vi "Counter - Continuous Output.vi"() -> ()   [LabVIEW 2012, in "Waveform.lvclass"]
doc: "This example demonstrates how to continuously generate digital pulses using a counter output."
uses:
  Waveform.lvclass
  <vilib>/Utility/error.llb/DialogType.ctl
  <vilib>/DAQmx/write.llb/DAQmx Write (Analog Wfm 1Chan NSamp).vi
  <vilib>/DAQmx/create/channels.llb/DAQmx Create Channel (CO-Pulse Generation-Frequency).vi
  <vilib>/DAQmx/configure/timing.llb/DAQmx Timing (Implicit).vi
  <vilib>/DAQmx/create/channels.llb/DAQmx Create Channel (AO-Voltage-Basic).vi
  <vilib>/DAQmx/configure/timing.llb/DAQmx Timing (Sample Clock).vi
  <vilib>/DAQmx/configure/trigger.llb/DAQmx Start Trigger (Digital Edge).vi
  <vilib>/DAQmx/miscellaneous.llb/DAQmx Fill In Error Info.vi
  <resource>/objmgr/daqmx.rc
  <vilib>/measure/NI_MABase.lvlib
panel:
  in  "Amplitude":dbl=1.0 format="%0.2p"
  in  "Signal Type":T1(ring)
  in  "HSYNC":i32=1000
  in  "Frame Rate":dbl=10000.0 caption="frame Rate" format="%0.2f"
  in  "Minimum Value":dbl=-10.0 format="%0.2f"
  in  "Maximum Value":dbl=10.0 format="%0.2f"
  in  "Physical Channels":tag="Dev1/ao0"
  in  "error in":errorcluster
  out "Actual Duty Cycle":dbl
  out "Actual Frequency":dbl
  in  "Duty Cycle":dbl=0.5 format="%.6f"
  in  "Frequency":dbl=1.0 format="%.6f"
  in  "Output Terminal":tag="/Dev1/PFI12"
  in  "Trigger Type":T2(tab)
  in  "Edge":i32(ring)=10280 items=["Rising"=10280, "Falling"=10171]
  in  "Digital Trigger Source":tag
  in  "Pause When":i32(ring)=10192 items=["High"=10192, "Low"=10214]
  in  "Pause Trigger Source":tag
  in  "Stop":bool
  in  "Counter":tag="Dev1/ctr0"
  # "Channel Settings"
  # "Trigger Settings"
  # "To configure and use a trigger you must have the necessary tab selected above."
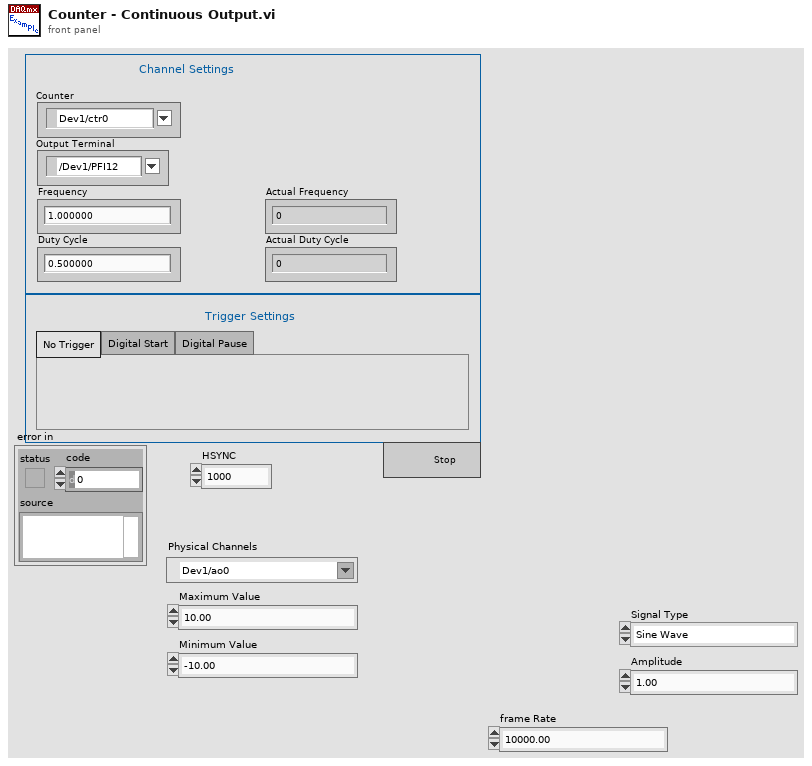
[diagram p1: front panel]
types:
  T1 = enum16{"Sine Wave", "Triangle Wave", "Square Wave", "Sawtooth Wave"}
  T2 = enum32{"No Trigger", "Digital Start", "Digital Pause"}
  T3 = typedef "DialogType.ctl" = u16
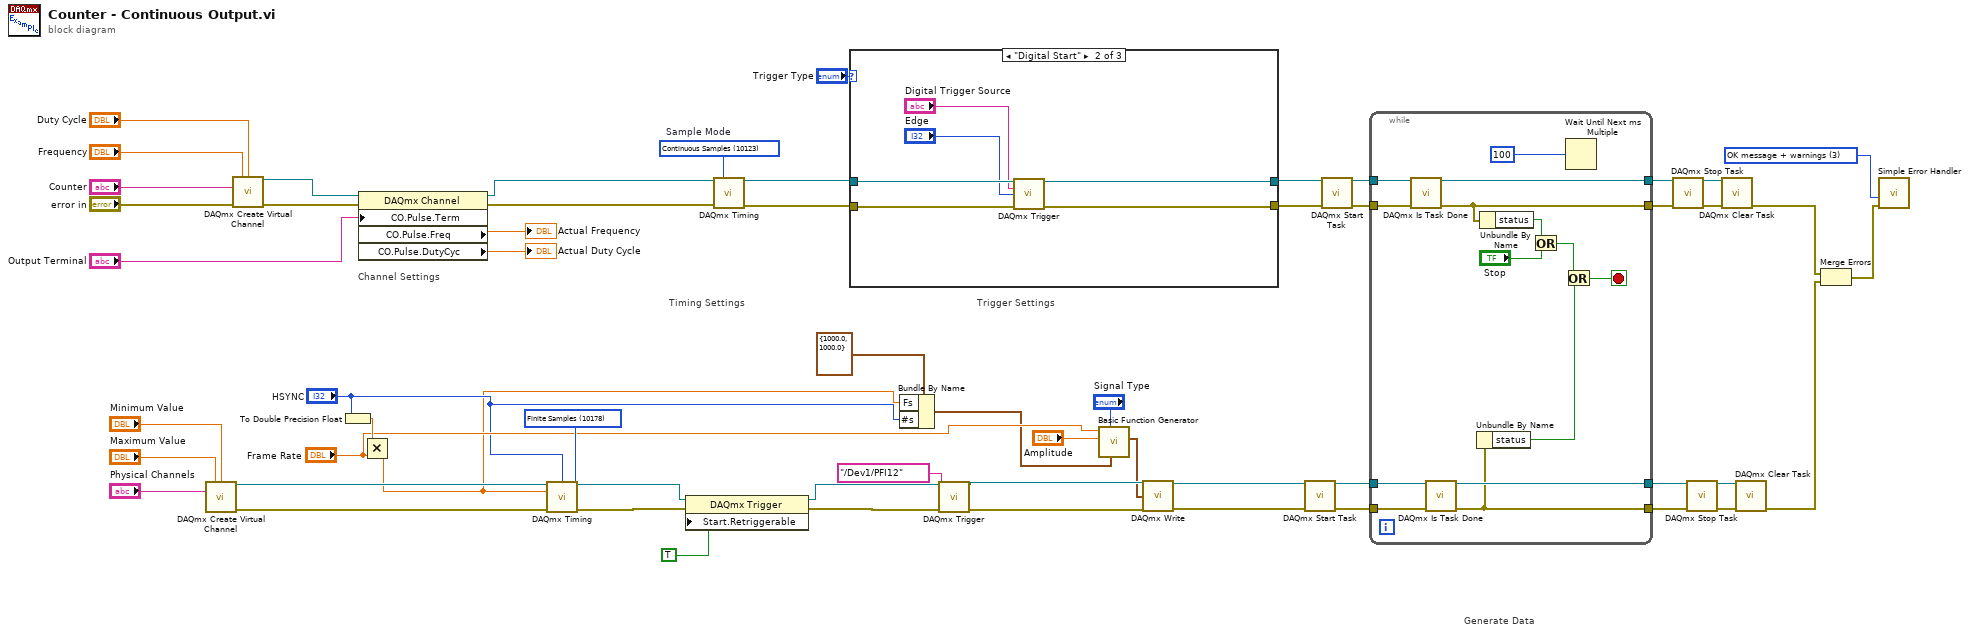
[diagram p0: block diagram]
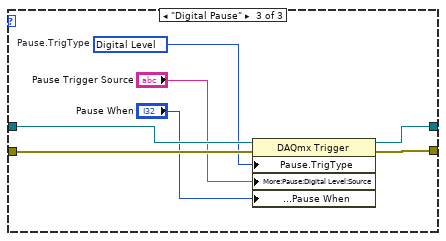
[diagram p3: hidden frame]
diagram:
  w29 = 10178 items=["Finite Samples"=10178, "Continuous Samples"=10123] ("sample mode")
  w36 = T3 3 items=["no dialog", "OK message", "continue or stop message", "OK message + warnings", "continue/stop + warnings"] ("type of dialog (OK msg:1)")
  w58 = 10123 items=["Finite Samples"=10178, "Continuous Samples"=10123, "Hardware Timed Single Point"=12522]  # Sample Mode
  # "Generate Data"
  # "Trigger Settings"
  # "Timing Settings"
  # "Channel Settings"
  n1 = call-poly <vilib>:"DAQmx Create Virtual Channel.vi"("maximum value"="Maximum Value", "minimum value"="Minimum Value", "physical channels"="Physical Channels") -> ("task out"=w32:refnum<k21>, "error out"=w28:errorcluster)  [unwired: 11 in]
  n2 = call-poly <vilib>:"DAQmx Create Virtual Channel.vi"("frequency"="Frequency", "duty cycle"="Duty Cycle", "counter"="Counter", "error in"="error in") -> ("task out"=w49:refnum<k21>, "error out"=w48:errorcluster)  [unwired: 10 in]
  n3 = To Double Precision Float(number="HSYNC") -> (double precision float=w33:dbl)
  n4 = property class="DAQmx Channel"(reference=w49, error in=w48, "CO.Pulse.Term"="Output Terminal") -> (reference out=w45:refnum<k21>, error out=w46:errorcluster, "CO.Pulse.Freq"=→"Actual Frequency":dbl, "CO.Pulse.DutyCyc"=→"Actual Duty Cycle":dbl)
  n5 = Multiply(x=w33, y="Frame Rate") -> (x*y=w7:dbl)
  n6 = call-poly <vilib>:"DAQmx Timing.vi"("task/channels in"=w32, "sample mode"=w29, "samples per channel"="HSYNC", "rate"=w7, "error in"=w28) -> ("task out"=w4:refnum<k21>, "error out"=w2:errorcluster)  [unwired: 9 in]
  n7 = property class="DAQmx Trigger"(reference=w4, error in=w2, "Start.Retriggerable"=TRUE) -> (reference out=w3:refnum<k21>, error out=w1:errorcluster)
  n8 = call-poly <vilib>:"DAQmx Timing.vi"("task/channels in"=w45, "sample mode"=w58, "error in"=w46) -> ("task out"=w53:refnum<k21>, "error out"=w52:errorcluster)  [unwired: 11 in]
  n9 = case shown="\"Digital Start\"" "Trigger Type" {
    tunnel: w53 -> [w60 w66 w73]
    tunnel: w52 -> [w59 w65 w70]
    tunnel: [w60 w64 w72] -> w50
    tunnel: [w59 w63 w71] -> w51
    frame "No Trigger", Default {
    }
    frame "Digital Start" {
      n10 = call-poly <vilib>:"DAQmx Trigger.vi"("task/channels in"=w66, "source"="Digital Trigger Source", "edge"="Edge", "error in"=w65) -> ("task out"=w64:refnum<k21>, "error out"=w63:errorcluster)  [unwired: 10 in]
    }
    frame "Digital Pause" {
      w69 = 10152 items=["Analog Level"=10101, "Analog Window"=10103, "Digital Level"=10152, "Digital Pattern"=10398, "None"=10230]  # Pause.TrigType
      n11 = property class="DAQmx Trigger"(reference=w73, error in=w70, "Pause.TrigType"=w69, "More:Pause:Digital Level:Source"="Pause Trigger Source", "More:Pause:Digital Level:Pause When"="Pause When") -> (reference out=w72:refnum<k21>, error out=w71:errorcluster)
    }
  }
  n12 = Bundle By Name(cluster=cluster{"Fs":dbl, "#s":dbl} {"Fs"=1000.0, "#s"=1000.0} ("sampling info"), "Fs"=w7, "#s"="HSYNC") -> (w6:cluster{"Fs":dbl, "#s":dbl})
  n13 = call-poly <vilib>:"DAQmx Trigger.vi"("task/channels in"=w3, "source"=tag "/Dev1/PFI12", "error in"=w1) -> ("task out"=w24:refnum<k21>, "error out"=w23:errorcluster)  [unwired: 11 in]
  n14 = call <vilib>:"Basic Function Generator.vi"("sampling info"=w6, "signal type"="Signal Type", "amplitude"="Amplitude", "frequency"="Frame Rate") -> ("signal out"=w22:waveform(dbl))  [unwired: 5 in, 2 out]
  n15 = call-poly <vilib>:"DAQmx Write.vi"("task/channels in"=w24, "data"=w22, "error in"=w23) -> ("task out"=w21:refnum<k21>, "error out"=w20:errorcluster)  [unwired: 10 in, 1 out]
  n16 = call <vilib>:"DAQmx Start Task.vi"("task/channels in"=w21, "error in"=w20) -> ("task out"=w19:refnum<k21>, "error out"=w18:errorcluster)  [unwired: 12 in]
  n17 = call <vilib>:"DAQmx Start Task.vi"("task/channels in"=w50, "error in"=w51) -> ("task out"=w57:refnum<k21>, "error out"=w56:errorcluster)  [unwired: 12 in]
  n18 = while {
    tunnel: w57 -> [w87]
    tunnel: w56 -> [w86]
    tunnel: [w84] -> w37
    tunnel: [w85] -> w38
    tunnel: w19 -> [w80]
    tunnel: w18 -> [w79]
    tunnel: [w78] -> w15
    tunnel: [w74] -> w14
    stop <- w75 stop-if-true
    n19 = call <vilib>:"DAQmx Is Task Done.vi"("task/channels in"=w87, "error in"=w86) -> ("task out"=w85:refnum<k21>, "error out"=w84:errorcluster)  [unwired: 11 in, 1 out]
    n20 = call <vilib>:"DAQmx Is Task Done.vi"("task/channels in"=w80, "error in"=w79) -> ("task out"=w78:refnum<k21>, "error out"=w74:errorcluster)  [unwired: 11 in, 1 out]
    n21 = Unbundle By Name(w74) -> ("status"=w77:bool)
    n22 = Unbundle By Name(w84) -> ("status"=w83:bool)
    n23 = Or(x=w83, y="Stop") -> (x .or. y?=w76:bool)
    n24 = Or(x=w76, y=w77) -> (x .or. y?=w75:bool)
    n25 = Wait Until Next ms Multiple(millisecond multiple=u32 100) -> ()  [unwired: 1 out]
  }
  n26 = call <vilib>:"DAQmx Stop Task.vi"("task/channels in"=w38, "error in"=w37) -> ("task out"=w40:refnum<k21>, "error out"=w39:errorcluster)  [unwired: 12 in]
  n27 = call <vilib>:"DAQmx Stop Task.vi"("task/channels in"=w15, "error in"=w14) -> ("task out"=w17:refnum<k21>, "error out"=w16:errorcluster)  [unwired: 12 in]
  n28 = call <vilib>:"DAQmx Clear Task.vi"("task in"=w40, "error in"=w39) -> ("error out"=w12:errorcluster)  [unwired: 13 in]
  n29 = call <vilib>:"DAQmx Clear Task.vi"("task in"=w17, "error in"=w16) -> ("error out"=w13:errorcluster)  [unwired: 13 in]
  n30 = Merge Errors(w12, w13) -> (w11:errorcluster)
  n31 = call <vilib>:"Simple Error Handler.vi"("type of dialog (OK msg:1)"=w36, "error in (no error)"=w11) -> ()  [unwired: 3 in, 5 out]
